vi "Disabled Property Panel.vi"() -> ()   [LabVIEW 2020, in "Property Panel.lvlib"]
uses:
  Property Panel.lvlib
panel:
  in  "Disabled Property":T1(ring)
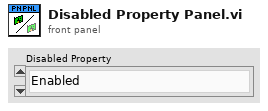
[diagram p1: front panel]
types:
  T1 = enum8{"Enabled", "Disabled", "Disabled and Grayed Out"}
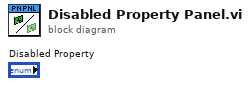
[diagram p0: block diagram]
diagram:
